vi "VCuarzo.vi"(1 "VISA resource name":refnum<visa-resource-name>="COM1") -> (0 "RATE":dbl=-0.02)   [LabVIEW 2011]
uses:
  <vilib>/Instr/_visa.llb/VISA Configure Serial Port (Instr).vi
panel:
  in  "read 2":bool=TRUE
  in  "write 2":bool=TRUE
  out "bytes read 2":u32=11
  out "read string 2":string="!*A-0.02 ,€"
  in  "?":dbl
  out "?":string="-0.02"
  in  "RUTA":path=path "c:/pru.txt"
  in  "flow control":u16(ring) items=["None"=0, "XON/XOFF"=1, "RTS/CTS"=2, "DTR/DSR"=4]
  in  "stop bits":u16(ring)=10 items=["1.0"=10, "1.5"=15, "2.0"=20]
  in  "parity":u16(ring) items=["None", "Odd", "Even", "Mark", "Space"]
  in  "data bits":u16=8 min=5 max=8 step=1
  in  "baud rate":u32=9600
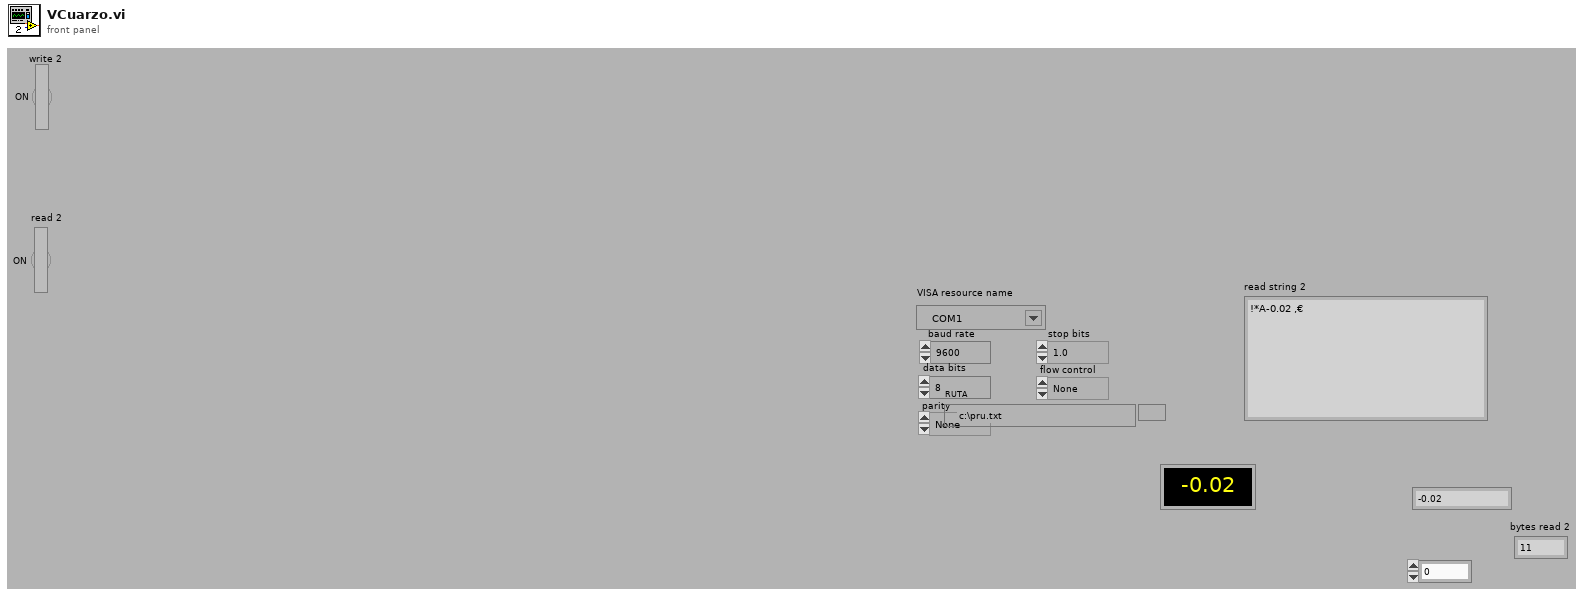
[diagram p1: front panel]
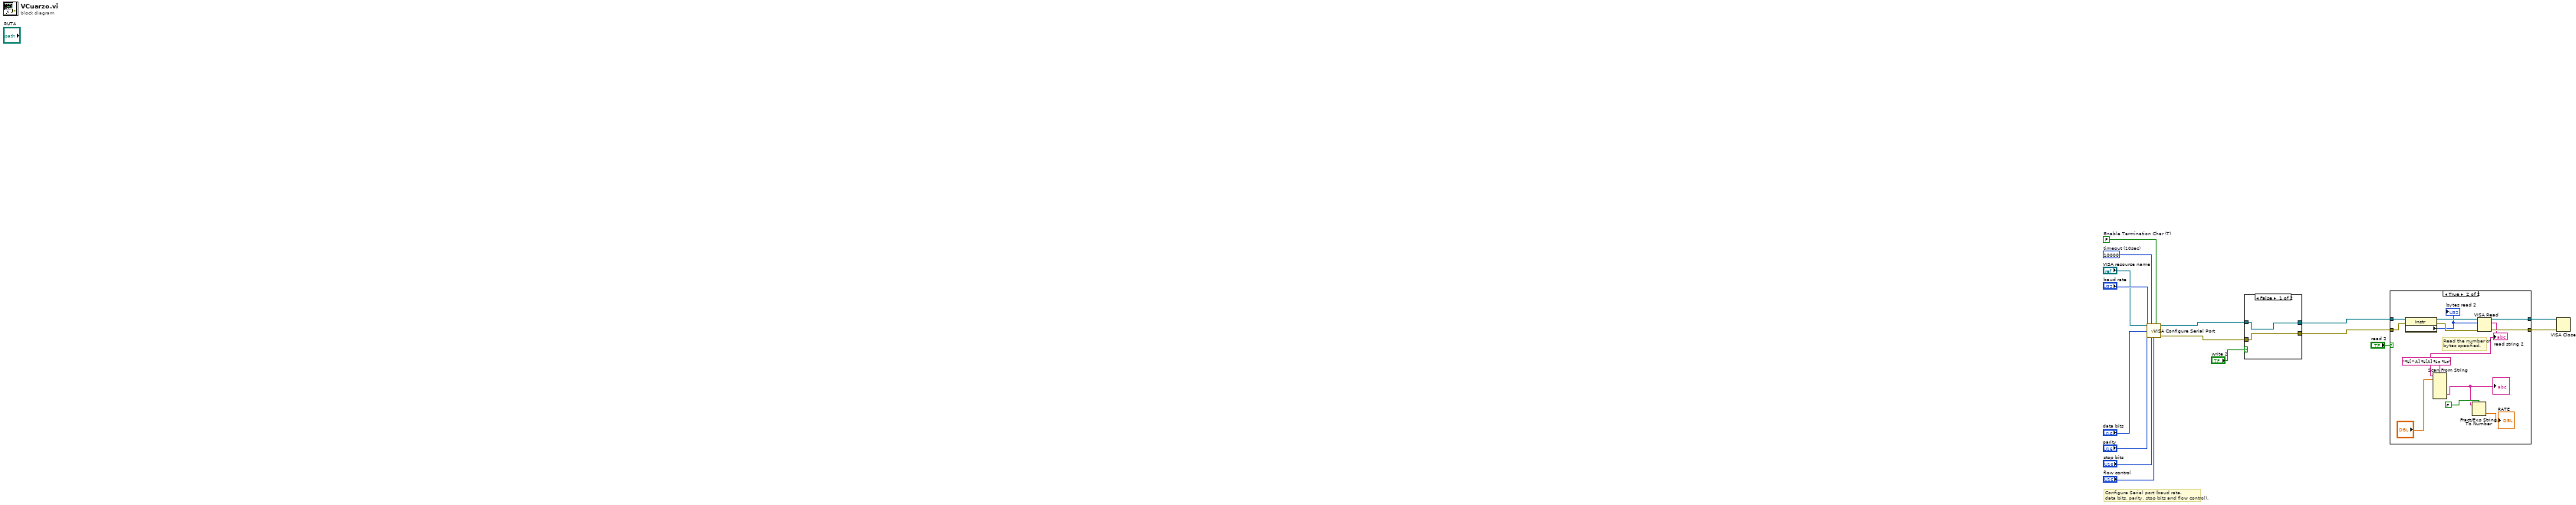
[diagram p0: block diagram]
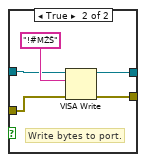
[diagram p2: hidden frame]
diagram:
  w12 = FALSE  # Enable Termination Char (T)
  w11 = u32 10000  # timeout (10sec)
  # "Configure Serial port (baud rate,\ndata bits, parity, stop bits and flow control)."
  n1 = call-poly "VISA Configure Serial Port"("VISA resource name"="VISA resource name", "timeout (10sec)"=w11, "Enable Termination\nChar (T)"=w12, "baud rate (9600)"="baud rate", "data bits (8)"="data bits", "parity (0:none)"="parity", "stop bits (10: 1 bit)"="stop bits", "flow control (0:none)"="flow control") -> ("error out"=w2:errorcluster)  [unwired: 6 in, 1 out]
  n2 = case shown="False" "write 2" {
    tunnel: [w16 w22] -> w3
    tunnel: [w17 w21] -> w4
    tunnel: w2 -> [w16 w19]
    tunnel: "VISA resource name" -> [w17 w18]
    frame False {
    }
    frame True {
      # "Write bytes to port."
      n3 = VISA Write(VISA resource name=w18, write buffer="!#MŽŠ", error in (no error)=w19) -> (VISA resource name out=w21:refnum<visa-resource-name>, error out=w22:errorcluster)  [unwired: 1 out]
    }
  }
  n4 = case shown="True" "read 2" {
    tunnel: w3 -> [w24 w33]
    tunnel: [w24 w37] -> w6
    tunnel: [w23 w36] -> w7
    tunnel: w4 -> [w23 w35]
    frame False {
    }
    frame True {
      # "Read the number of bytes specified."
      n5 = property class="Instr"(reference=w35, error in=w33) -> (reference out=w34:refnum<visa-resource-name>, error out=w32:errorcluster, "Serial Settings:Number of Bytes at Serial Port"=w31:u32)
      "bytes read 2" <- w31
      n6 = VISA Read(VISA resource name=w34, byte count=w31, error in (no error)=w32) -> (VISA resource name out=w36:refnum<visa-resource-name>, read buffer=w30:string, error out=w37:errorcluster)  [unwired: 1 out]
      "read string 2" <- w30
      n7 = Scan From String(format string="%[^A] %[A] %s %s", input string=w30, initial scan location="?") -> (output 3=w25:string)  [unwired: 8 in, 3 out]
      "?" <- w25
      n8 = Fract/Exp String To Number(use system decimal point (T)=FALSE, string=w25) -> (number=→"RATE":dbl)  [unwired: 2 in, 1 out]
    }
  }
  n9 = VISA Close(VISA resource name=w7, error in (no error)=w6) -> ()  [unwired: 1 out]
